vi "Load-libraries.vi"(8 "error in (no error)":errorcluster, 11 "SM1000-control in":T1) -> (0 "error out":errorcluster, 1 "Loaded?":bool, 3 "SM1000-control out":T1)   [LabVIEW 2013, in "MaterialCharacterization.lvlib" / "MC-SM1000.lvclass"]
uses:
  MC-SM1000.lvclass
  Object-reference.ctl
  C:/Users/vangeste/Desktop/2015-06-02 - SLM - MAIF/HC-HardwareCharacterization/Sources/SM1000/LECBroadcast.dll
  HC-HardwareCharacterization/Sources/SM1000/LECBroadcast.dll
  C:/Users/vangeste/Desktop/2015-06-02 - SLM - MAIF/HC-HardwareCharacterization/Sources/SM1000/LECSession.dll
  HC-HardwareCharacterization/Sources/SM1000/LECSession.dll
  MC-SM1000.lvclass/MC-SM1000.ctl
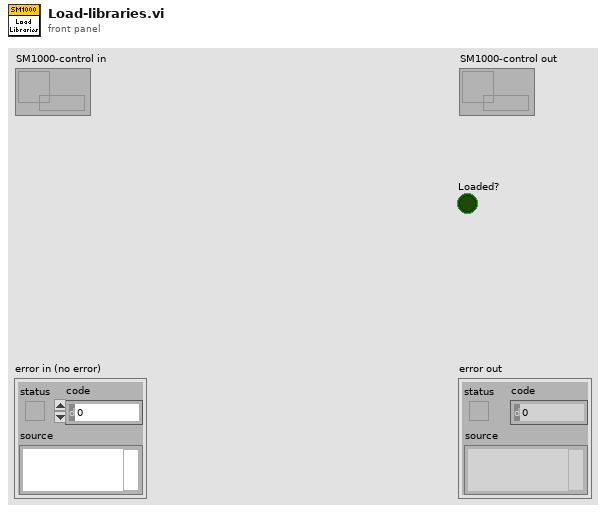
[diagram p1: front panel]
types:
  T1 = typedef "MaterialCharacterization.lvlib/MC-SM1000.lvclass/Object-reference.ctl" = refnum<data-value>
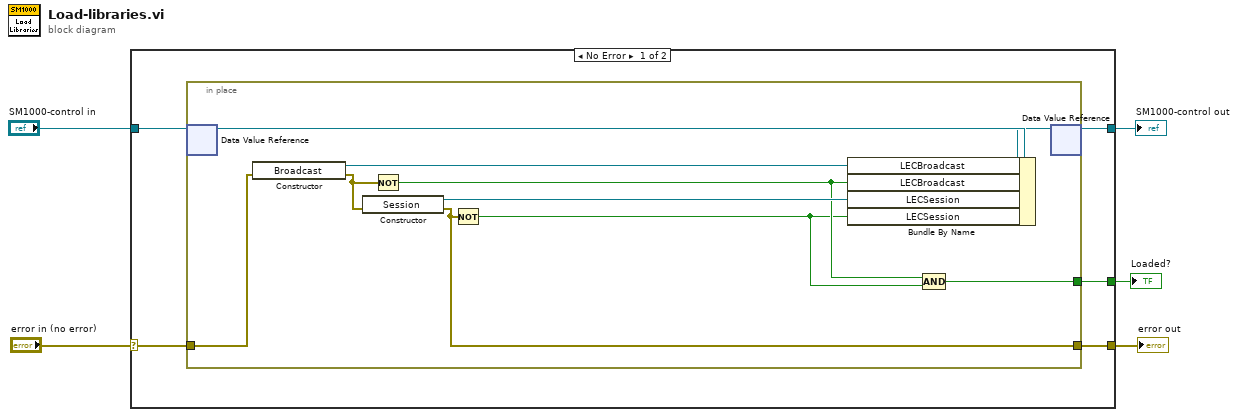
[diagram p0: block diagram]
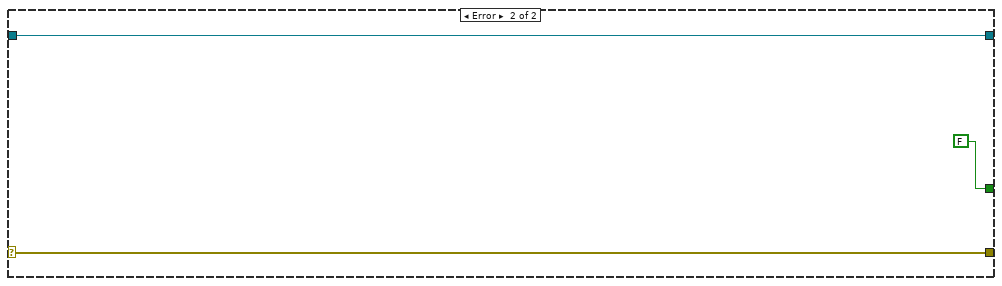
[diagram p2: hidden frame]
diagram:
  n1 = case shown="No Error" "error in (no error)" {
    selector: "error in (no error)" -> [w8 w23]
    tunnel: [w7 w23] -> w4
    tunnel: [w9 w22] -> w2
    tunnel: "SM1000-control in" -> [w10 w22]
    tunnel: [w6 FALSE] -> w1
    frame No Error {
      n2 = in-place {
        in-place-border: w8 -> [w18]
        in-place-border: [w14] -> w7
        in-place-border: [w11] -> w6
        n3 = in-place-dvr #1(w10) -> (w20:refnum<class "MC-SM1000.lvclass">)  [unwired: 1 out]
        n4 = constructor class="Broadcast"(error in=w18) -> (reference out=w17:refnum<k24>, error out=w16:errorcluster)  [unwired: 2 in, 1 out]
        n5 = constructor class="Session"(error in=w16) -> (reference out=w15:refnum<k24>, error out=w14:errorcluster)  [unwired: 2 in, 1 out]
        n6 = Not(x=w16) -> (.not. x?=w13:bool)
        n7 = Not(x=w14) -> (.not. x?=w12:bool)
        n8 = Bundle By Name(cluster=w20, "LECBroadcast"=w17, "LECBroadcast"=w13, "LECSession"=w15, "LECSession"=w12) -> (w19:refnum<class "MC-SM1000.lvclass">)
        n9 = Compound Arithmetic op=AND(w13, w12) -> (w11:bool)
        n10 = in-place-dvr #1(w19) -> (w9:T1)  [unwired: 1 out]
      }
    }
    frame Error {
    }
  }
  "error out" <- w4
  "SM1000-control out" <- w2
  "Loaded?" <- w1
